vi "Coordinates to Point.vi"(3 "Coordinates":cdb) -> (1 "point":cluster{"x":dbl, "y":dbl})   [LabVIEW 2020, in "AoC 2022.lvlib"]
uses:
  AoC 2022.lvlib
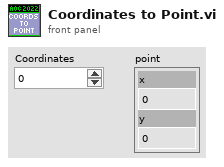
[diagram p1: front panel]
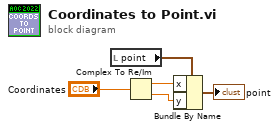
[diagram p0: block diagram]
diagram:
  n1 = local read "point"() -> (w1:cluster{"x":dbl, "y":dbl})
  n2 = Complex To Re/Im(x + iy="Coordinates") -> (x=w3:dbl, y=w4:dbl)
  n3 = Bundle By Name(cluster=w1, "x"=w3, "y"=w4) -> (→"point":cluster{"x":dbl, "y":dbl})
